vi "Optimized Call Command.vi"(11 "Command":T1) -> (0 "error out":errorcluster)   [LabVIEW 2025]
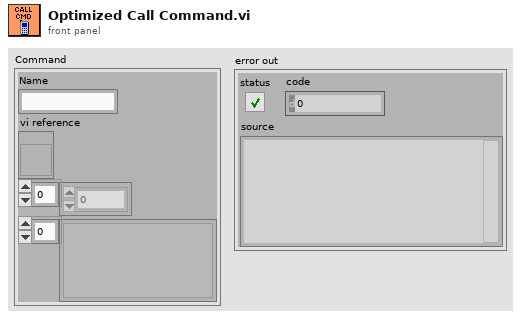
[diagram p1: front panel]
types:
  T1 = cluster{"Name":string, "vi reference":refnum<vi>, i32[], variant[]}
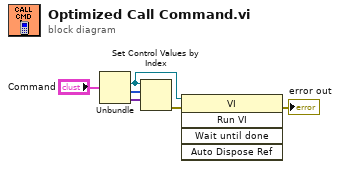
[diagram p0: block diagram]
diagram:
  n1 = Unbundle("Command") -> ("vi reference"=w1:refnum<vi>, w4:i32[], w3:variant[])  [unwired: 1 out]
  n2 = Set Control Values by Index(0:w1, 1:w4, 2:w3) -> (11:w5:errorcluster)  [unwired: 1 in]
  n3 = invoke class="VI" method="Run VI"(reference=w1, error in=w5) -> (error out=→"error out":errorcluster)  [unwired: 3 in, 4 out]
